vi "Set_Unit.vi"(2 "error in":errorcluster, 3 "Unit":string(combo), 4 "VISA arduino in":refnum<visa-resource-name>) -> (0 "error out":errorcluster, 1 "VISA arduino out":refnum<visa-resource-name>)   [LabVIEW 2021]
uses:
  Delay_Global.vi
  <vilib>/Utility/error.llb/Error Cluster From Error Code.vi
  <vilib>/ErrorRing/Error Ring.xnode
panel:
  out "delay":u32
  # "Private"
  # "Public"
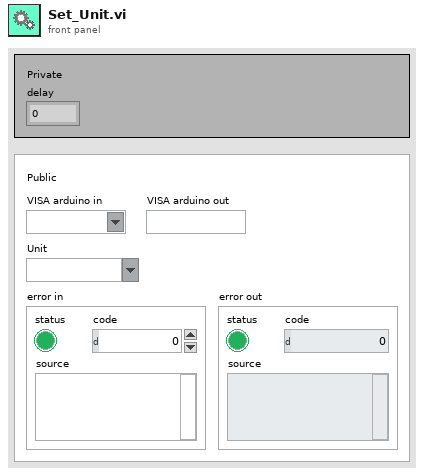
[diagram p1: front panel]
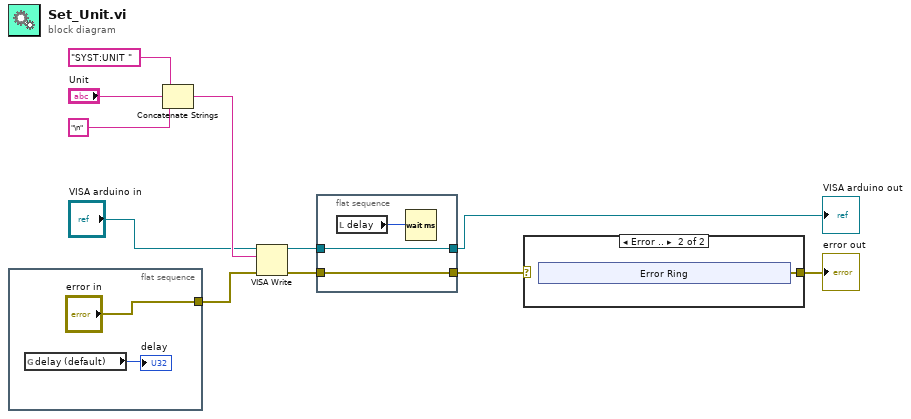
[diagram p0: block diagram]
diagram:
  n1 = flat-sequence {
    tunnel: ["error in"] -> w1
    frame #0 {
      n2 = global read "Delay_Global.vi" "delay (default)"() -> (→"delay":u32)
    }
  }
  n3 = Concatenate Strings("SYST:UNIT ", "Unit", "\n" ("string")) -> (w3:string)
  n4 = VISA Write(VISA resource name="VISA arduino in", write buffer=w3, error in (no error)=w1) -> (VISA resource name out=w10:refnum<visa-resource-name>, error out=w9:errorcluster)  [unwired: 1 out]
  n5 = flat-sequence {
    tunnel: [w16] -> w6
    tunnel: w10 -> [w16]
    tunnel: [w15] -> w11
    tunnel: w9 -> [w15]
    frame #0 {
      n6 = local read "delay"() -> (w14:u32)
      n7 = Wait (ms)(milliseconds to wait=w14) -> ()  [unwired: 1 out]
    }
  }
  n8 = case shown="Error .." w11 {
    selector: w11 -> [w17 _]
    tunnel: [w17 w18] -> w7
    frame No Error {
    }
    frame Error {
      n9 = xnode "Error Ring"() -> ("error out"=w18:errorcluster)
    }
  }
  "error out" <- w7
  "VISA arduino out" <- w6
